vi "ContinuousDBMeasure.vi"() -> ()   [LabVIEW 2017]
panel:
  out "Power":dbl
  in  "stop (F)":bool
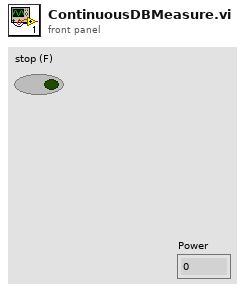
[diagram p1: front panel]
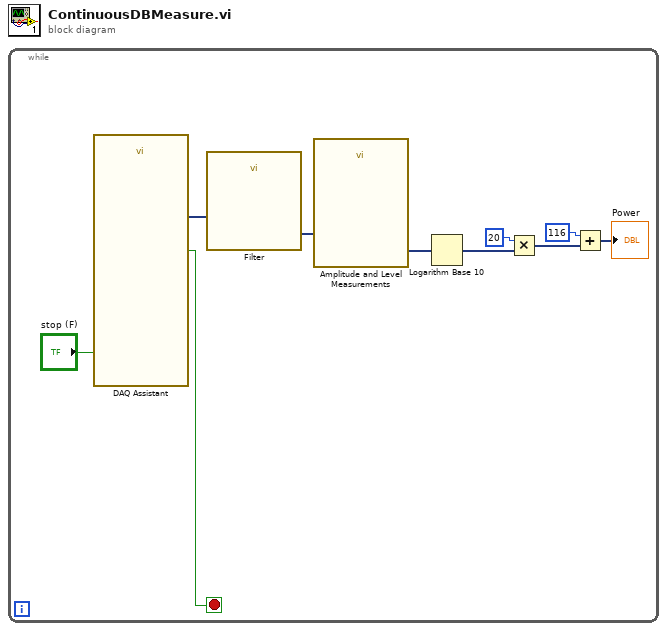
[diagram p0: block diagram]
diagram:
  n1 = while {
    stop <- w10 stop-if-true
    n2 = call "DAQ Assistant"("stop (F)"="stop (F)") -> ("data"=w8:dynamicdata, "stopped"=w10:bool)  [unwired: 15 in, 2 out]
    n3 = call "Filter"("Signal"=w8) -> ("Filtered Signal"=w7:dynamicdata)  [unwired: 9 in, 1 out]
    n4 = call "Amplitude and Level Measurements"("Signals"=w7) -> ("RMS"=w5:dynamicdata)  [unwired: 13 in, 1 out]
    n5 = Logarithm Base 10(1:w5) -> (0:w4:dynamicdata)
    n6 = Multiply(x=20, y=w4) -> (x*y=w3:dynamicdata)
    n7 = Add(x=116, y=w3) -> (x+y=→"Power":dynamicdata)
  }
